vi "TableEntry.vi"(8 "error in (no error)":errorcluster) -> (0 "error out":errorcluster, 1 "Dwell Time @ SP (sec) 2":u32 step=1 format="%.0f sec", 2 "Cooling rate (°C/min) 2":dbl=0.01 min=0.01 max=5.0 step=0.01 format="%.2g °C/min", 3 "SP (°C) 2":dbl min=-50.0 max=50.0 step=0.1 format="%.1g °C", 4 "Add Entry Pressed?":bool)   [LabVIEW 2013]
doc: "Use this template to build a VI to use as a subVI."
panel:
  in  "Get Focus":u32 step=1 format="%.0f sec"
  in  "Cancel Button":bool
  in  "Add Entry Button":bool
  in  "Dwell Time @ SP (sec)":u32 step=1 format="%.0f sec"
  in  "Cooling rate (°C/min)":dbl=0.01 min=0.01 max=50.0 step=0.01 format="%.2g °C/min"
  in  "SP (°C)":dbl min=-100.0 max=50.0 step=0.1 format="%.1g °C"
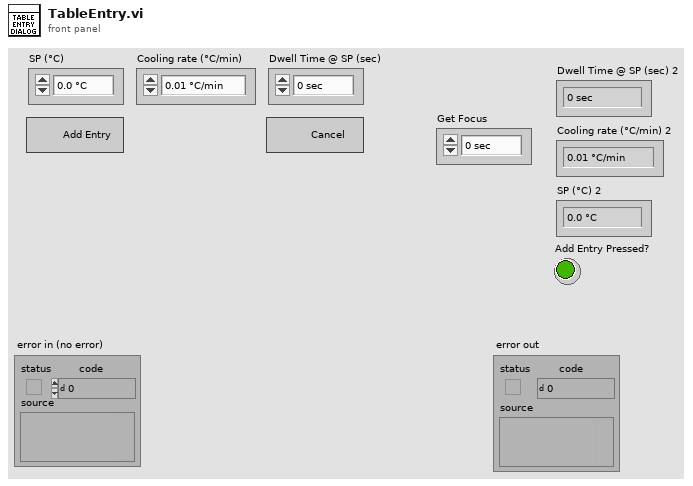
[diagram p1: front panel]
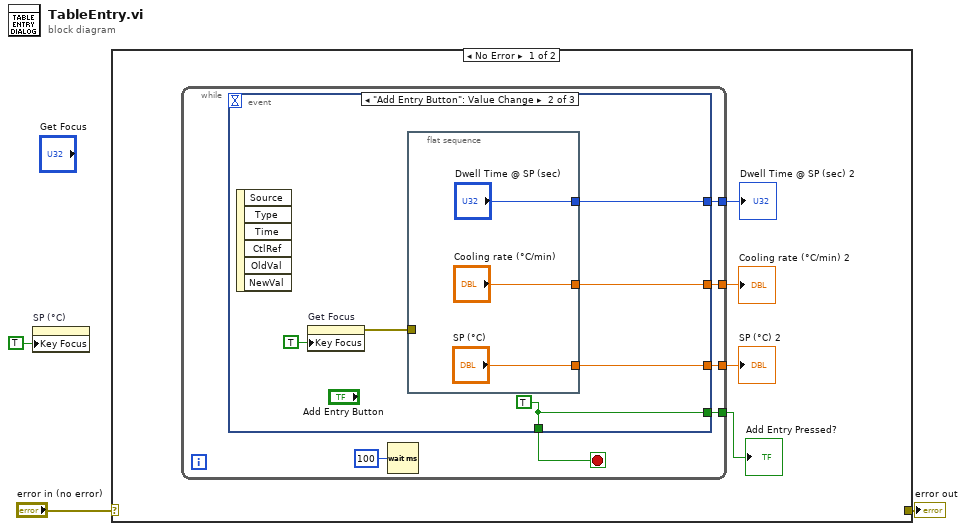
[diagram p0: block diagram]
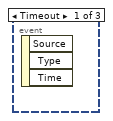
[diagram p2: hidden frame]
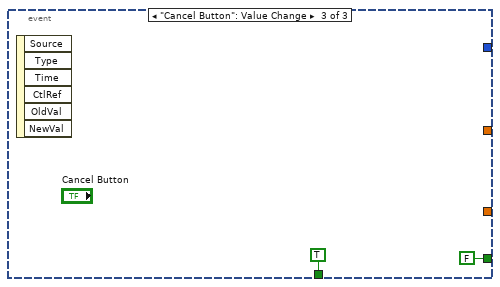
[diagram p3: hidden frame]
diagram:
  n1 = property on="SP (°C)" class="DigNum (strict)"("Key Focus"=TRUE) -> ()  [unwired: 2 in, 2 out]
  n2 = case shown="No Error" "error in (no error)" {
    selector: "error in (no error)" -> [_ w25]
    tunnel: [_ w25] -> w2
    frame No Error {
      n3 = while {
        tunnel: [w12] -> w7
        tunnel: [w11] -> w6
        tunnel: [w10] -> w5
        tunnel: [w9] -> w4
        stop <- w13 stop-if-true
        n4 = event shown="[1] \"Add Entry Button\": Value Change" {
          selector: _ -> [_ _ _]
          dyn-events: _ -> [_ _ _]
          timeout: _ -> [_ _ _]
          tunnel: [_ w16 TRUE] -> w13
          tunnel: [_ w19 _] -> w12
          tunnel: [_ w18 _] -> w11
          tunnel: [_ w17 _] -> w10
          tunnel: [_ w16 FALSE] -> w9
          event Timeout {
            n5 = event-data() -> ()  [unwired: 1 in, 3 out]
          }
          event "Add Entry Button": Value Change {
            w16 = TRUE
            n6 = event-data() -> ()  [unwired: 1 in, 6 out]
            n7 = property on="Get Focus" class="DigNum (strict)"("Key Focus"=TRUE) -> (error out=w14:errorcluster)  [unwired: 2 in, 1 out]
            n8 = flat-sequence {
              tunnel: ["Dwell Time @ SP (sec)"] -> w19
              tunnel: ["Cooling rate (°C/min)"] -> w18
              tunnel: ["SP (°C)"] -> w17
              tunnel: w14 -> [_]
              frame #0 {
              }
            }
          }
          event "Cancel Button": Value Change {
            n9 = event-data() -> ()  [unwired: 1 in, 6 out]
          }
        }
        n10 = Wait (ms)(milliseconds to wait=u32 100) -> ()  [unwired: 1 out]
      }
      "Cooling rate (°C/min) 2" <- w6
      "Dwell Time @ SP (sec) 2" <- w7
      "SP (°C) 2" <- w5
      "Add Entry Pressed?" <- w4
    }
    frame Error {
    }
  }
  "error out" <- w2
